vi "EXA_logEvent_SettingVersions.vi"(8 "error in (no error)":errorcluster, 11 "logevent_SettingVersions_Ctl":T1) -> (0 "error out":errorcluster, 2 "function return":i32, 3 "logevent_SettingVersions_Ctl out":T1)   [LabVIEW 2016, in "SALLV_EXA.lvlib"]
doc: "int EXA_shm_logEvent_SettingVersionsLV(EXA_logevent_SettingVersionsLV *logevent_SettingVersions_Ctl );"
uses:
  SALLV_EXA.lvlib
  DataTypes/logevent_SettingVersions.ctl
  SALLV_EXA.so
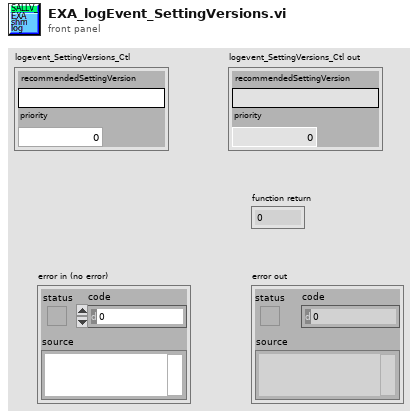
[diagram p1: front panel]
types:
  T1 = typedef "SALLV_EXA.lvlib/logevent_SettingVersions.ctl" = cluster{"recommendedSettingVersion":string, "priority":i32}
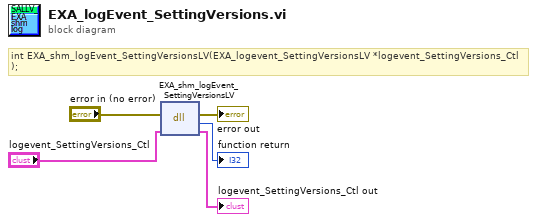
[diagram p0: block diagram]
diagram:
  # "int EXA_shm_logEvent_SettingVersionsLV(EXA_logevent_SettingVersionsLV *logevent_SettingVersions_Ctl );"
  n1 = dll-call lib="home/hsundar/TCS/updated_EXA/SALLV_EXA.*" fn="EXA_shm_logEvent_SettingVersionsLV"(error in="error in (no error)", "logevent_SettingVersions_Ctl"="logevent_SettingVersions_Ctl") -> (error out=→"error out":errorcluster, →"function return":i32, "logevent_SettingVersions_Ctl"=→"logevent_SettingVersions_Ctl out":T1)  [unwired: 2 in, 1 out]
